vi "Inalfa SCU_Manual_LIN Message.vi"(0 "Choose Sequence":T1, 1 "LIN Device":T2={"Master Frame(3C)"="MasterReq\nSPA3414_ConfigurationsCMAGeely_CEMCALYPSOSDB34XX0Cfg_LIN3_190709_", "Slave Frame(3D)"="SlaveResp\nSPA3414_ConfigurationsCMAGeely_CEMCALYPSOSDB34XX0Cfg_LIN3_190709_", "Request Schedule"="CEMLIN3DiagRequestSchedule\nSPA3414_ConfigurationsCMAGeely_CEMCALYPSOSDB34XX0Cfg_LIN3_190709_", "Response Schedule"="CEMLIN3DiagResponseSchedule\nSPA3414_ConfigurationsCMAGeely_CEMCALYPSOSDB34XX0Cfg_LIN3_190709_", "Frame Write SCU"="", "Frame Read SCU"="", "LIN Name"=""}, 2 "Position":u16, 3 "Vent Cycles":u16, 4 "Slide Cycles":u16, 5 "Tx":u8[][](array[numeric]) format="%02x", 6 "Only Tx":u8[][](array[numeric]) format="%02x", 7 "Rx":u8[](array[numeric]) format="%02x", 8 "String":string, 10 "NAD":u8=36 format="%.0x") -> (11 "glass position":u16, 12 "TxRx Data":string[][](array[string]), 13 "sunshade position":u16, 14 "Response Good?":bool, 15 "Software Level":string, 16 "Hardware Level":string, 17 "Calfile Level":string, 18 "Glass Slide Cycle":u16, 19 "Rx2":u8[](array[numeric]) format="%02x")   [LabVIEW 2018]
uses:
  LIN Device.ctl
  LIN sequence for self SCU.ctl
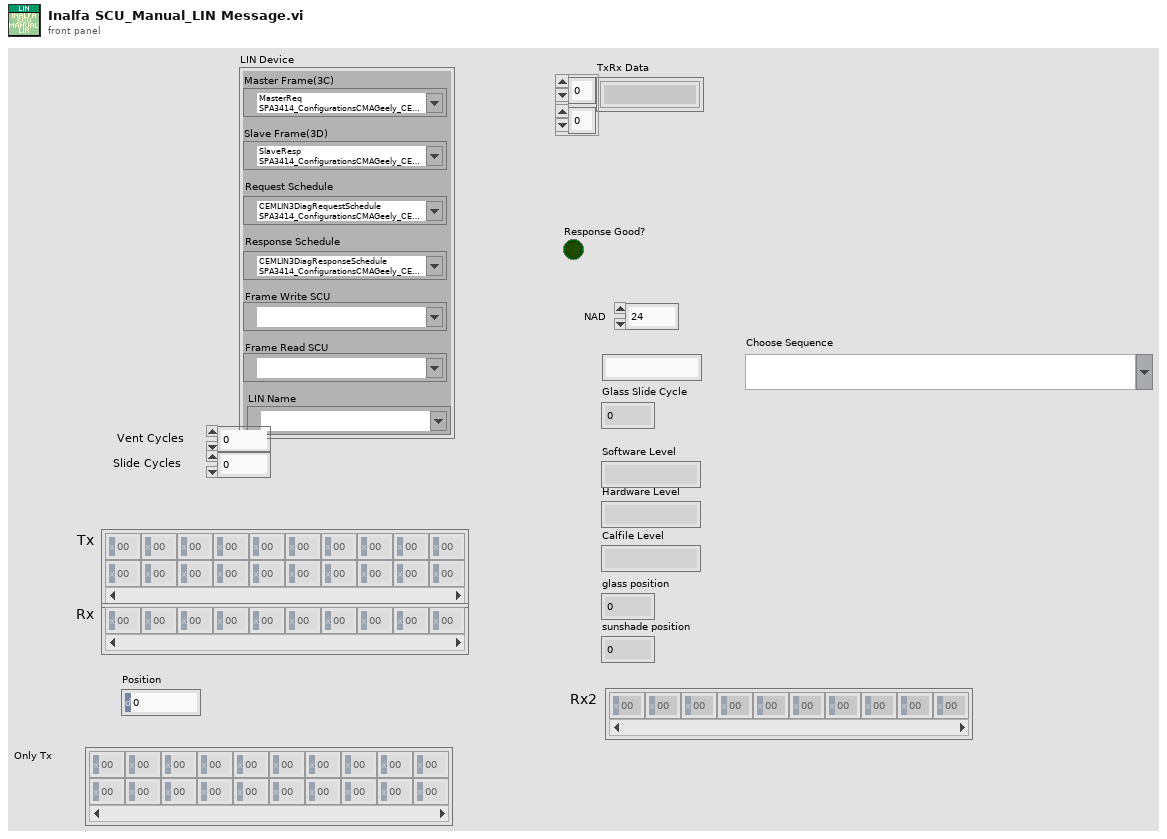
[diagram p1: front panel]
types:
  T1 = typedef "LIN sequence for self SCU.ctl" = string
  T2 = typedef "LIN Device.ctl" = cluster{"Master Frame(3C)":refnum<k21>, "Slave Frame(3D)":refnum<k21>, "Request Schedule":refnum<k21>, "Response Schedule":refnum<k21>, "Frame Write SCU":refnum<k21>, "Frame Read SCU":refnum<k21>, "LIN Name":refnum<k21>}
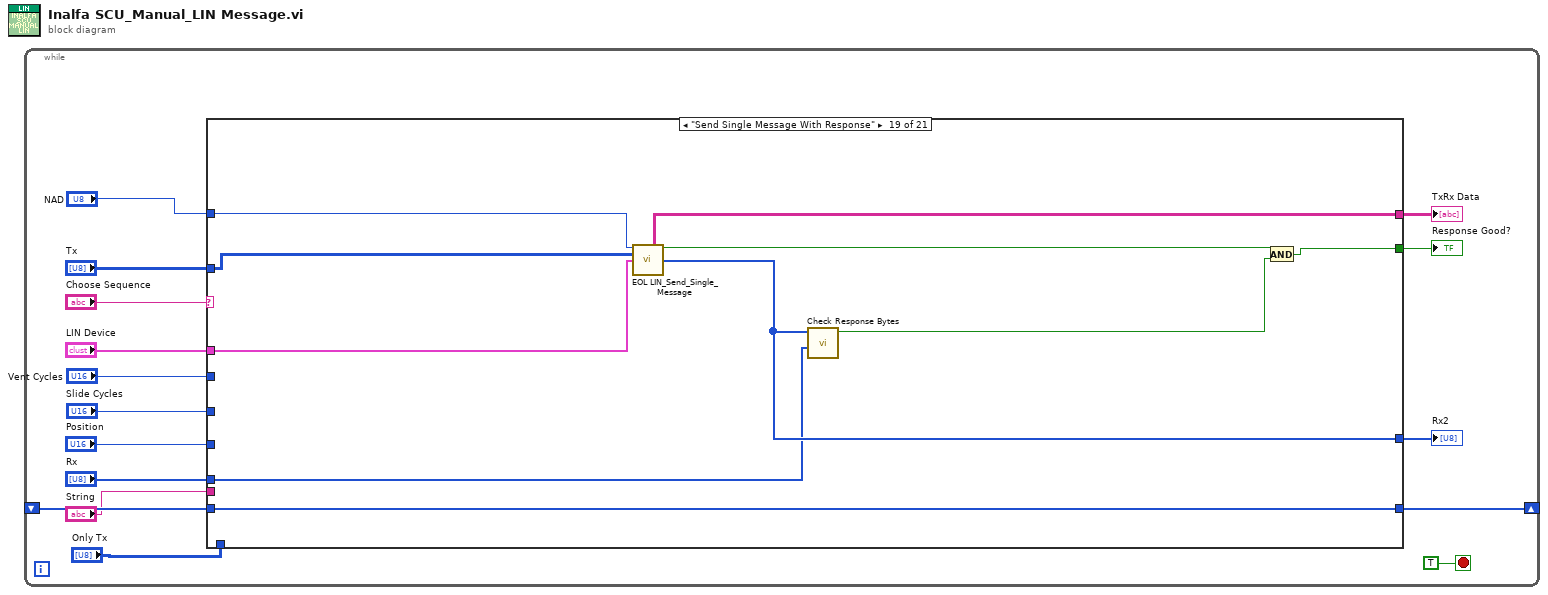
[diagram p0: block diagram]
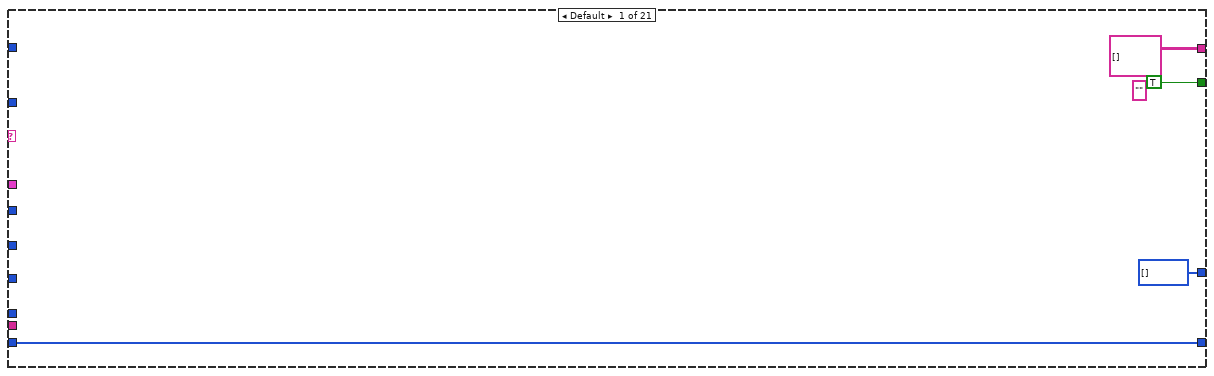
[diagram p2: hidden frame]
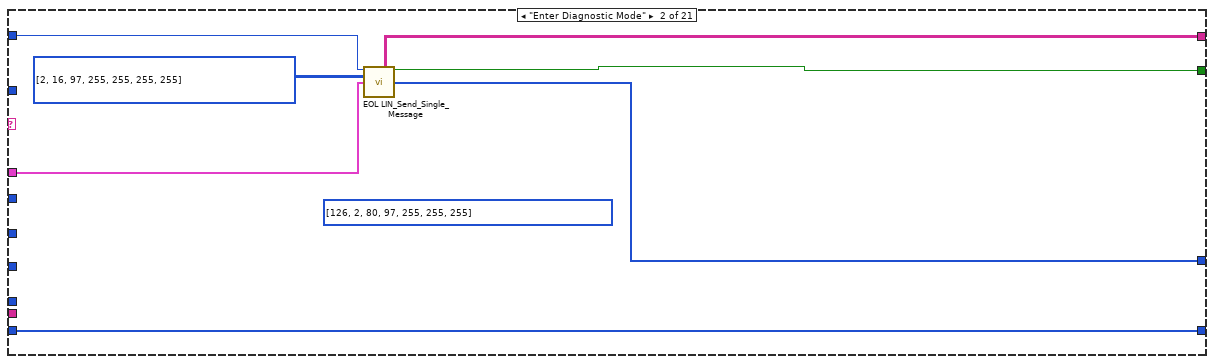
[diagram p3: hidden frame]
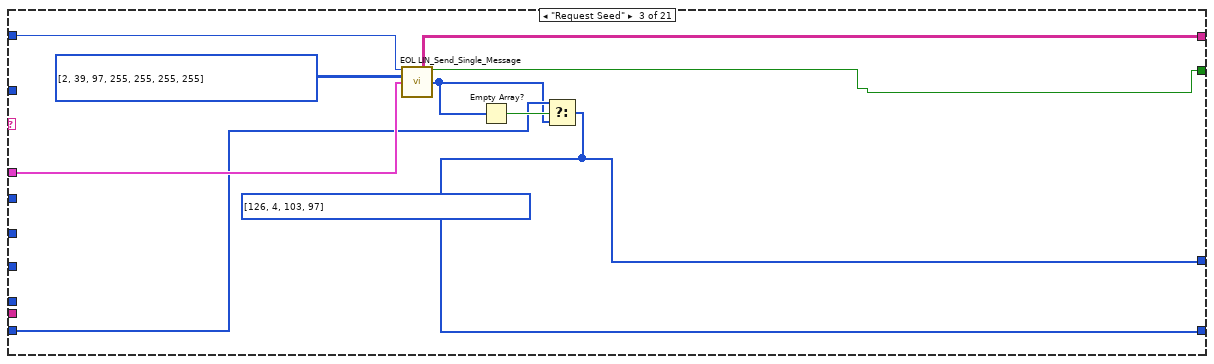
[diagram p4: hidden frame]
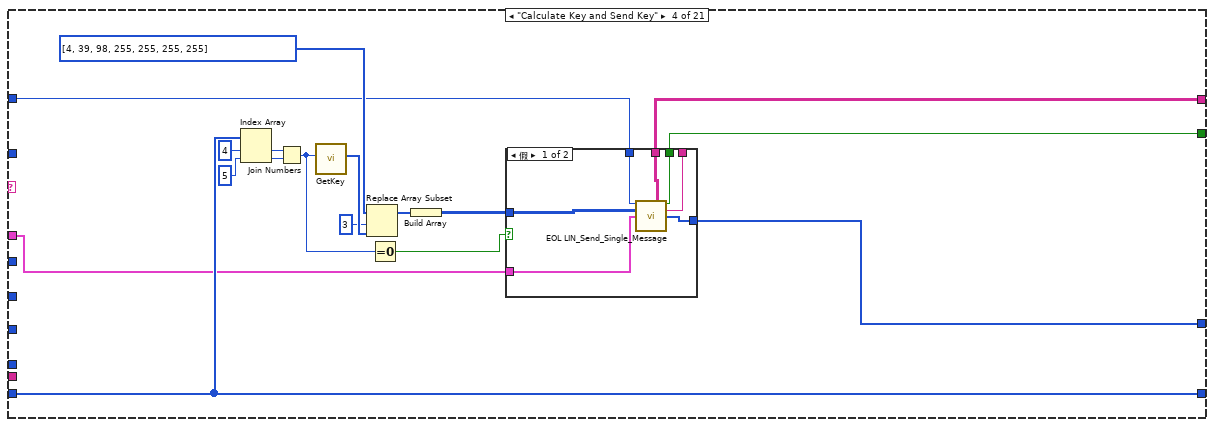
[diagram p5: hidden frame]
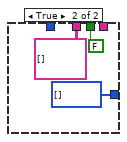
[diagram p6: hidden frame]
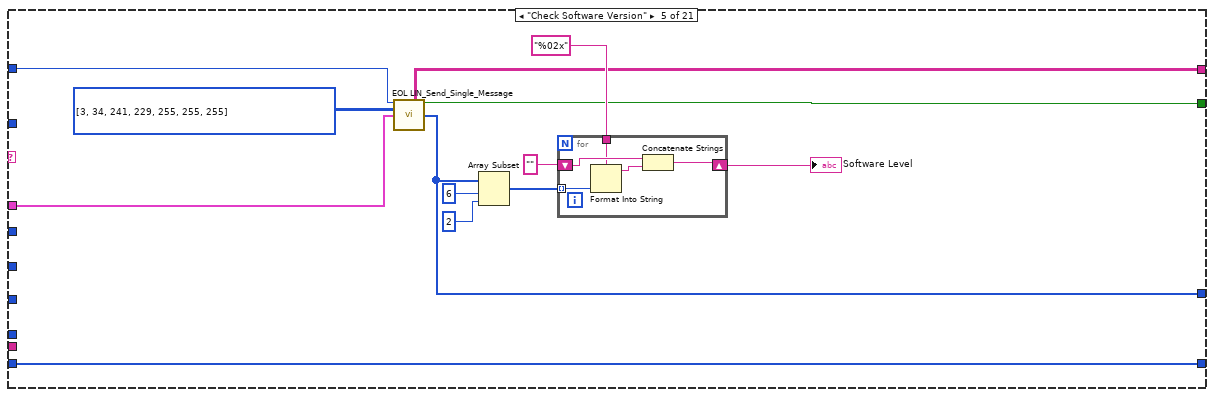
[diagram p7: hidden frame]
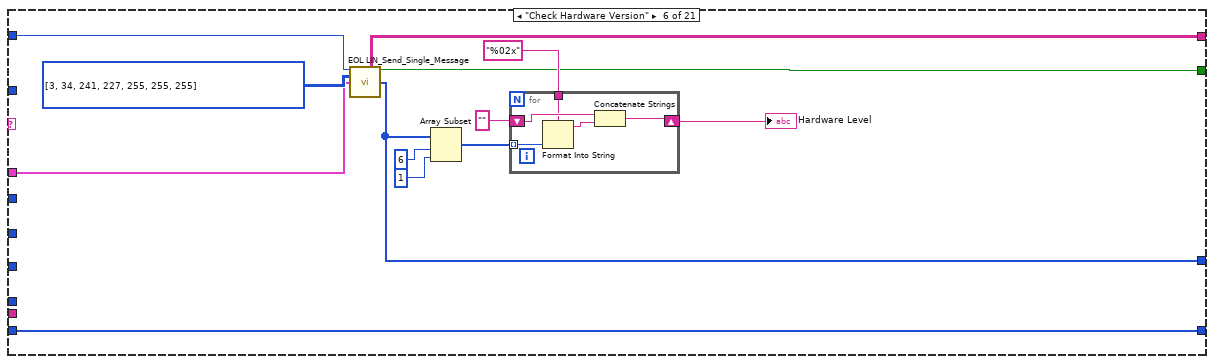
[diagram p8: hidden frame]
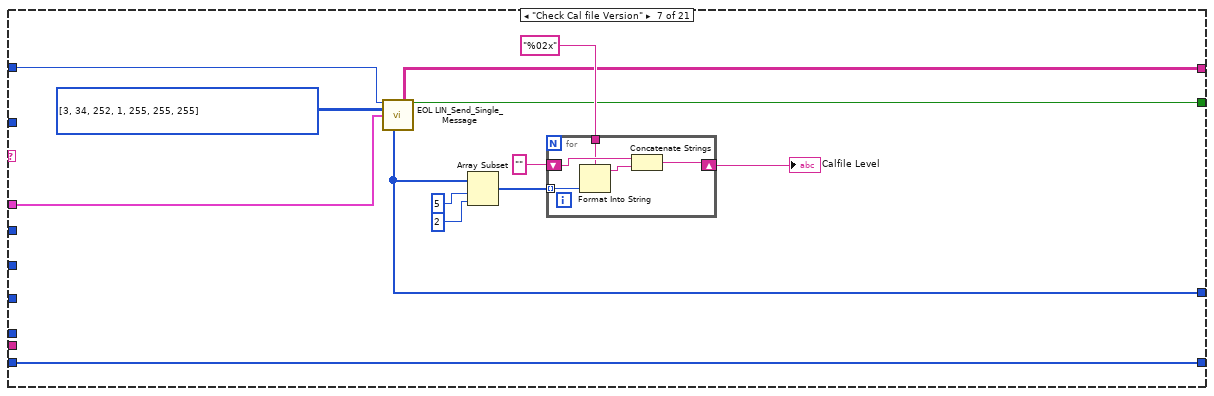
[diagram p9: hidden frame]
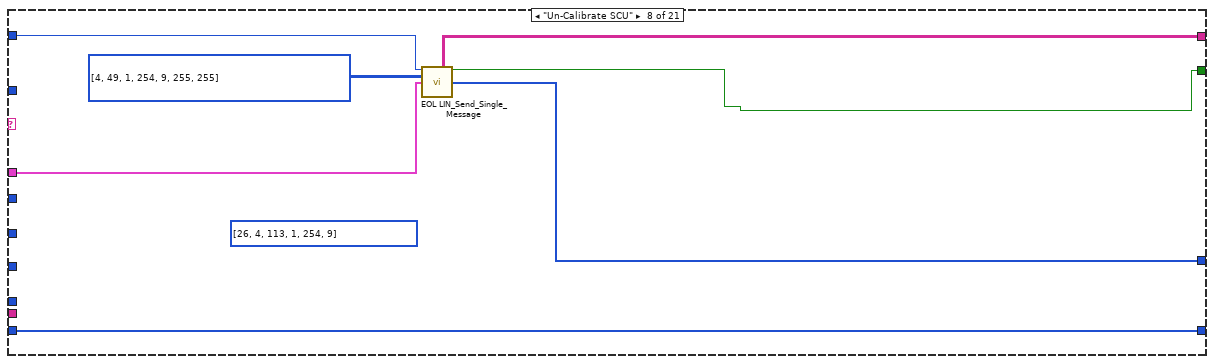
[diagram p10: hidden frame]
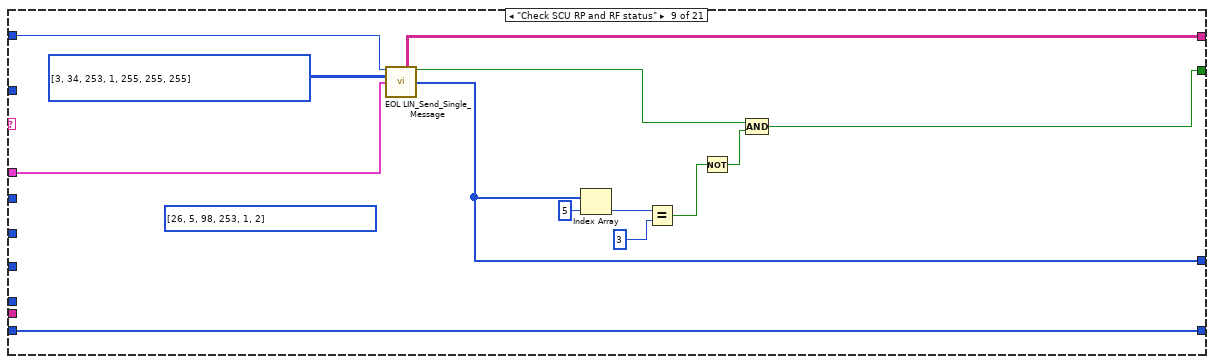
[diagram p11: hidden frame]
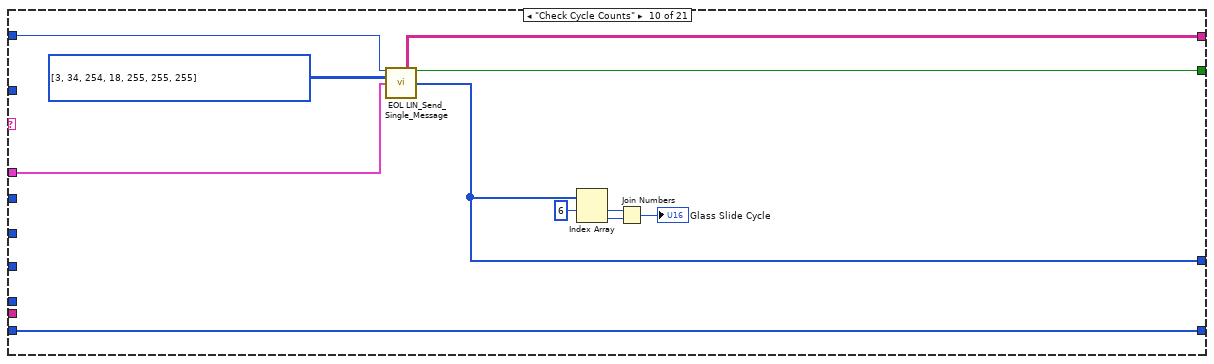
[diagram p12: hidden frame]
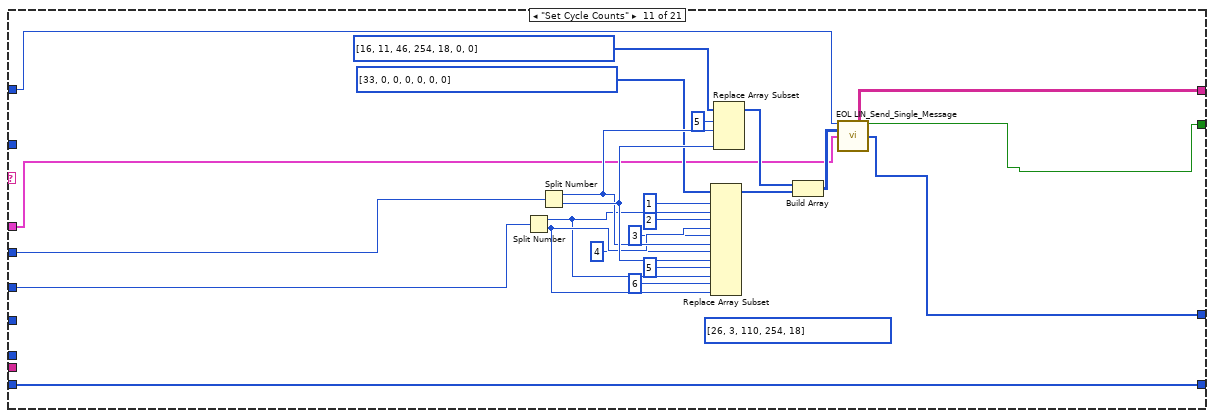
[diagram p13: hidden frame]
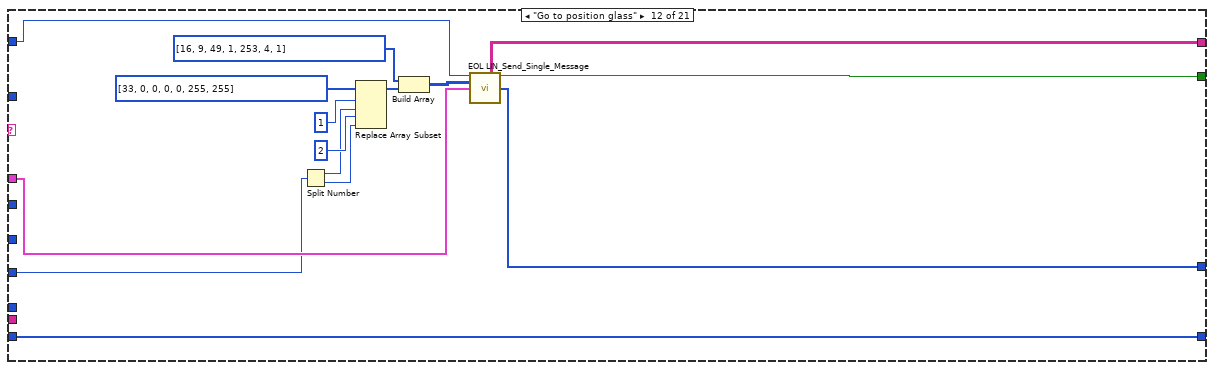
[diagram p14: hidden frame]
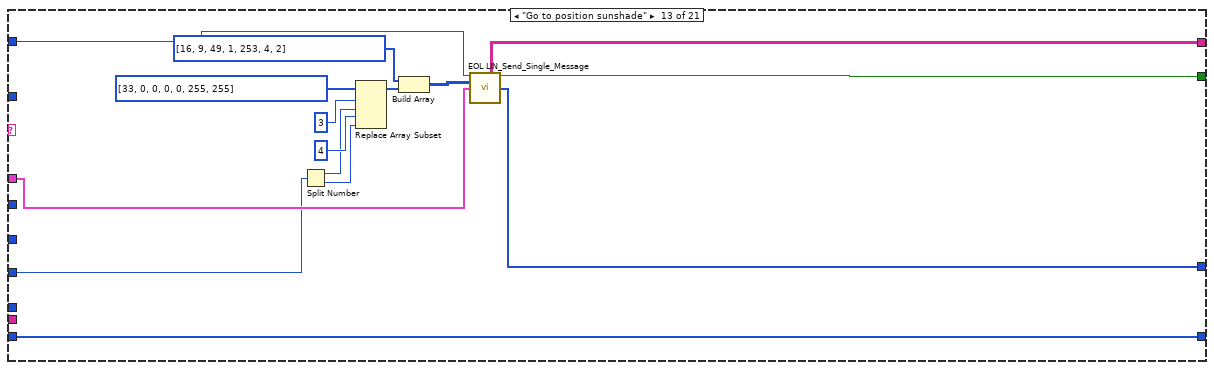
[diagram p15: hidden frame]
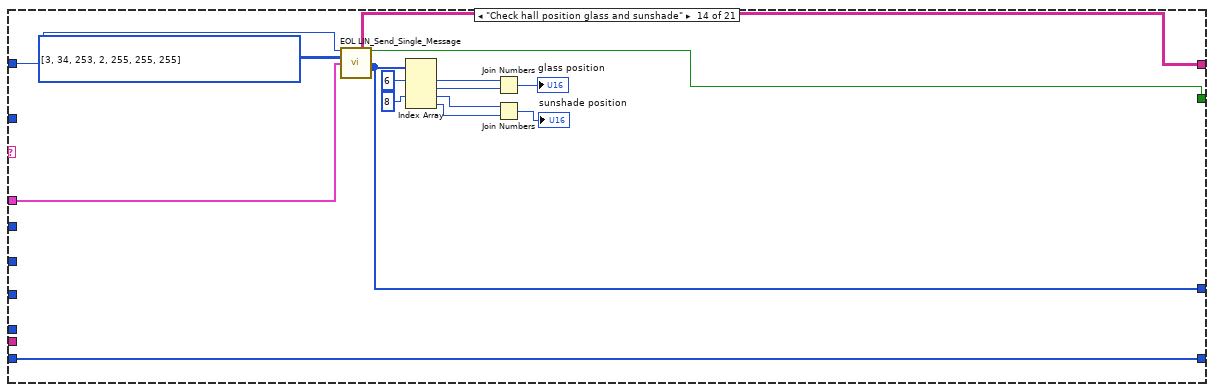
[diagram p16: hidden frame]
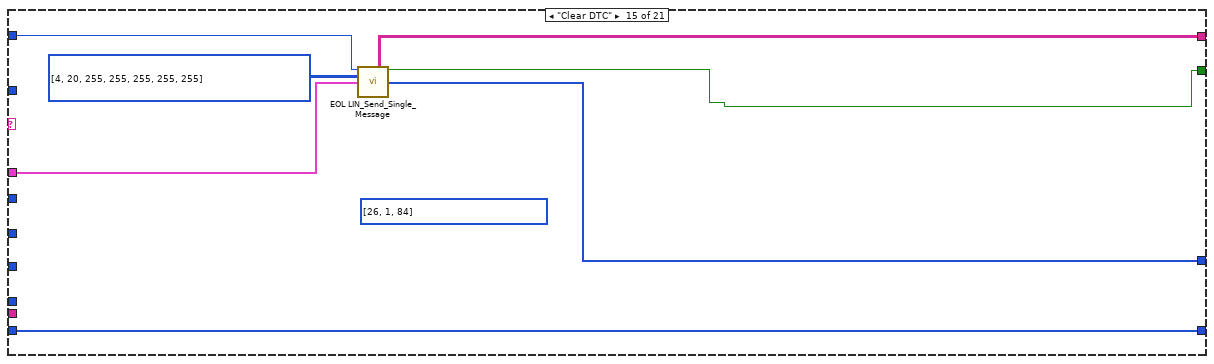
[diagram p17: hidden frame]
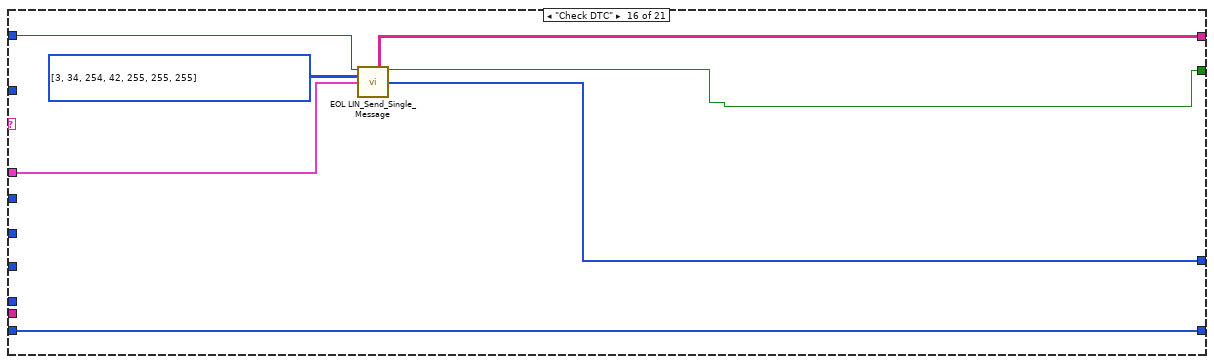
[diagram p18: hidden frame]
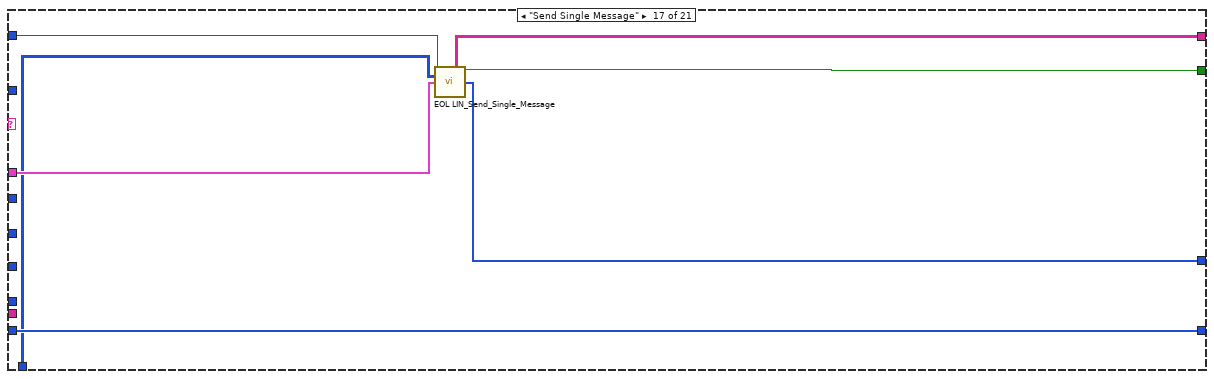
[diagram p19: hidden frame]
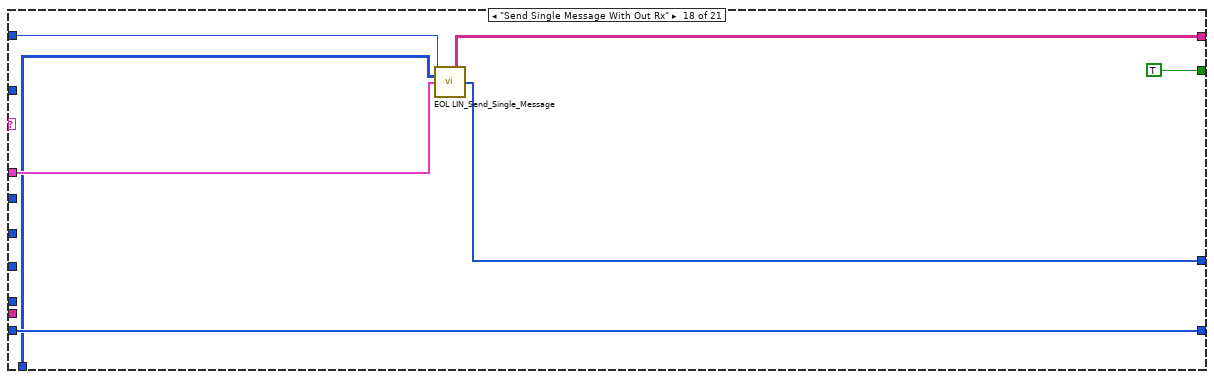
[diagram p20: hidden frame]
diagram:
  n1 = while {
    shift-right: [w12] -> _
    shift-left: _ -> [w11]
    stop <- TRUE stop-if-true
    n2 = case shown="\"Send Single Message With Response\"" "Choose Sequence" {
      tunnel: "LIN Device" -> [_ w26 w34 w39 w75 w87 w105 w123 w136 w147 w154 w176 w191 w208 w222 w229 w235 w242 w253 w265 w271]
      tunnel: [string[][] [] ("TxRx Data") w25 w35 w42 w69 w93 w107 w122 w135 w146 w156 w179 w194 w212 w223 w230 w238 w245 w255 w268 w274] -> w15
      tunnel: [TRUE ("Response Good?") w21 w28 w40 w65 w83 w101 w118 w132 w139 w149 w178 w193 w206 w218 w225 w237 TRUE ("Response Good?") w247 w267 w273] -> w14
      tunnel: [w18 w24 w31 w41 w68 w86 w104 w121 w134 w145 w155 w177 w192 w209 w221 w228 w236 w243 w254 w266 w272] -> w12
      tunnel: w11 -> [w18 w24 w32 w41 w68 w86 w104 w121 w134 w145 w155 w177 w192 w209 w221 w228 w236 w243 w254 w266 w272]
      tunnel: [u8[] [] ("Rx Message") w22 w31 w38 w67 w85 w103 w120 w126 w143 w153 w175 w190 w207 w220 w227 w234 w241 w251 w264 w270] -> w4
      tunnel: "Position" -> [_ _ _ _ _ _ _ _ _ _ _ w174 w189 _ _ _ _ _ _ _ _]
      tunnel: "Tx" -> [_ _ _ _ _ _ _ _ _ _ _ _ _ _ _ _ _ _ w252 _ _]
      tunnel: "Vent Cycles" -> [_ _ _ _ _ _ _ _ _ _ w152 _ _ _ _ _ _ _ _ _ _]
      tunnel: "Slide Cycles" -> [_ _ _ _ _ _ _ _ _ _ w151 _ _ _ _ _ _ _ _ _ _]
      tunnel: "Rx" -> [_ _ _ _ _ _ _ _ _ _ _ _ _ _ _ _ _ _ w250 _ _]
      tunnel: "Only Tx" -> [_ _ _ _ _ _ _ _ _ _ _ _ _ _ _ _ w233 w240 _ _ _]
      tunnel: "String" -> [_ _ _ _ _ _ _ _ _ _ _ _ _ _ _ _ _ _ _ w257 _]
      tunnel: "NAD" -> [_ w23 w29 w37 w64 w82 w100 w119 w125 w142 w150 w173 w188 w203 w219 w226 w232 w239 w246 w256 w269]
      frame Default {
        (unwired) "" ("spreadsheet string")
      }
      frame "Enter Diagnostic Mode" {
        (unwired) u8[] [126, 2, 80, 97, 255, 255, 255]
        n3 = call "EOL LIN_Send_Single_Message.vi"("NAD"=w23, "Tx Msg"=u8[][] [[2, 16, 97, 255, 255, 255, 255]], "LIN Device"=w26) -> ("TxRx Data"=w25:string[][], "Response Good?"=w21:bool, "Rx Msg"=w22:u8[])  [unwired: 8 in, 2 out]
      }
      frame "Request Seed" {
        (unwired) u8[] [126, 4, 103, 97]
        n4 = call "EOL LIN_Send_Single_Message.vi"("NAD"=w29, "Tx Msg"=u8[][] [[2, 39, 97, 255, 255, 255, 255]], "LIN Device"=w34) -> ("TxRx Data"=w35:string[][], "Response Good?"=w28:bool, "Rx Msg"=w30:u8[])  [unwired: 8 in, 2 out]
        n5 = Empty Array?(array=w30) -> (empty?=w33:bool)
        n6 = Select(t=w32, s=w33, f=w30) -> (s? t:f=w31:u8[])
      }
      frame "Calculate Key and Send Key" {
        n7 = Index Array(array=w41, index #1=4 ("index"), index #2=5 ("index")) -> (element #1=w51:u8, element #2=w50:u8)
        n8 = Join Numbers(hi=w51, lo=w50) -> ((hi.lo)=w45:u16)
        n9 = call "GetKey.vi"("x"=w45) -> ("KEY"=w49:u8[])  [unwired: 10 in]
        n10 = Replace Array Subset(array=u8[] [4, 39, 98, 255, 255, 255, 255], new element=w49, index=3) -> (w46:u8[])
        n11 = Equal To 0?(x=w45) -> (x = 0?=w43:bool)
        n12 = Build Array(w46) -> (w44:u8[][])
        n13 = case shown="假" w43 {
          tunnel: w44 -> [w60 _]
          tunnel: [w59 string[][] [] ("TxRx Data")] -> w42
          tunnel: [w58 FALSE ("Response Good?")] -> w40
          tunnel: [w57 _] -> _
          tunnel: w39 -> [w56 _]
          tunnel: [w55 u8[] [] ("Rx Message")] -> w38
          tunnel: w37 -> [w54 _]
          frame False {
            n14 = call "EOL LIN_Send_Single_Message.vi"("NAD"=w54, "Tx Msg"=w60, "LIN Device"=w56) -> ("TxRx Data"=w59:string[][], "Response Good?"=w58:bool, "spreadsheet string"=w57:string, "Rx Msg"=w55:u8[])  [unwired: 8 in, 1 out]
          }
          frame True {
          }
        }
      }
      frame "Check Software Version" {
        n15 = call "EOL LIN_Send_Single_Message.vi"("NAD"=w64, "Tx Msg"=u8[][] [[3, 34, 241, 229, 255, 255, 255]], "LIN Device"=w75) -> ("TxRx Data"=w69:string[][], "Response Good?"=w65:bool, "Rx Msg"=w67:u8[])  [unwired: 8 in, 2 out]
        n16 = Array Subset(array=w67, index=6, length=2) -> (w74:u8[])
        n17 = for {
          tunnel: w74 -> [w77] mode=indexing
          shift-right: [w80] -> w66
          shift-left: "" -> [w79]
          tunnel: "%02x" ("format string") -> [w78]
          n18 = Format Into String(format string=w78, w77) -> (resulting string=w81:string)  [unwired: 2 in, 1 out]
          n19 = Concatenate Strings(w79, w81) -> (w80:string)
        }
        "Software Level" <- w66
      }
      frame "Check Hardware Version" {
        n20 = call "EOL LIN_Send_Single_Message.vi"("NAD"=w82, "Tx Msg"=u8[][] [[3, 34, 241, 227, 255, 255, 255]], "LIN Device"=w87) -> ("TxRx Data"=w93:string[][], "Response Good?"=w83:bool, "Rx Msg"=w85:u8[])  [unwired: 8 in, 2 out]
        n21 = Array Subset(array=w85, index=6, length=1) -> (w92:u8[])
        n22 = for {
          tunnel: w92 -> [w95] mode=indexing
          shift-right: [w98] -> w84
          shift-left: "" -> [w97]
          tunnel: "%02x" ("format string") -> [w96]
          n23 = Format Into String(format string=w96, w95) -> (resulting string=w99:string)  [unwired: 2 in, 1 out]
          n24 = Concatenate Strings(w97, w99) -> (w98:string)
        }
        "Hardware Level" <- w84
      }
      frame "Check Cal file Version" {
        n25 = call "EOL LIN_Send_Single_Message.vi"("NAD"=w100, "Tx Msg"=u8[][] [[3, 34, 252, 1, 255, 255, 255]], "LIN Device"=w105) -> ("TxRx Data"=w107:string[][], "Response Good?"=w101:bool, "Rx Msg"=w103:u8[])  [unwired: 8 in, 2 out]
        n26 = Array Subset(array=w103, index=5, length=2) -> (w112:u8[])
        n27 = for {
          tunnel: w112 -> [w113] mode=indexing
          shift-right: [w116] -> w102
          shift-left: "" -> [w115]
          tunnel: "%02x" ("format string") -> [w114]
          n28 = Format Into String(format string=w114, w113) -> (resulting string=w117:string)  [unwired: 2 in, 1 out]
          n29 = Concatenate Strings(w115, w117) -> (w116:string)
        }
        "Calfile Level" <- w102
      }
      frame "Un-Calibrate SCU" {
        (unwired) u8[] [26, 4, 113, 1, 254, 9]
        n30 = call "EOL LIN_Send_Single_Message.vi"("NAD"=w119, "Tx Msg"=u8[][] [[4, 49, 1, 254, 9, 255, 255]], "LIN Device"=w123) -> ("TxRx Data"=w122:string[][], "Response Good?"=w118:bool, "Rx Msg"=w120:u8[])  [unwired: 8 in, 2 out]
      }
      frame "Check SCU RP and RF status" {
        (unwired) u8[] [26, 5, 98, 253, 1, 2]
        n31 = call "EOL LIN_Send_Single_Message.vi"("NAD"=w125, "Tx Msg"=u8[][] [[3, 34, 253, 1, 255, 255, 255]], "LIN Device"=w136) -> ("TxRx Data"=w135:string[][], "Response Good?"=w133:bool, "Rx Msg"=w126:u8[])  [unwired: 8 in, 2 out]
        n32 = Index Array(array=w126, index=5) -> (element=w130:u8)
        n33 = Equal?(x=w130, y=u8 3 ("element")) -> (x = y?=w128:bool)
        n34 = Not(x=w128) -> (.not. x?=w127:bool)
        n35 = Compound Arithmetic op=AND(w133, w127) -> (w132:bool)
      }
      frame "Check Cycle Counts" {
        n36 = call "EOL LIN_Send_Single_Message.vi"("NAD"=w142, "Tx Msg"=u8[][] [[3, 34, 254, 18, 255, 255, 255]], "LIN Device"=w147) -> ("TxRx Data"=w146:string[][], "Response Good?"=w139:bool, "Rx Msg"=w143:u8[])  [unwired: 8 in, 2 out]
        n37 = Index Array(array=w143, index #1=6 ("index")) -> (element #1=w141:u8, element #2=w140:u8)  [unwired: 1 in]
        n38 = Join Numbers(hi=w141, lo=w140) -> ((hi.lo)=→"Glass Slide Cycle":u16)
      }
      frame "Set Cycle Counts" {
        (unwired) u8[] [26, 3, 110, 254, 18]
        n39 = Split Number(x=w151) -> (hi(x)=w167:u8, lo(x)=w168:u8)
        n40 = Split Number(x=w152) -> (hi(x)=w169:u8, lo(x)=w170:u8)
        n41 = Replace Array Subset(array=u8[] [33, 0, 0, 0, 0, 0, 0] ("Frame payloads to queue"), new element #1=w167, index #1=1 ("索引"), new element #2=w168, index #2=2 ("索引"), new element #3=w169, index #3=3 ("索引"), new element #4=w170, index #4=4 ("索引"), new element #5=w167, index #5=5 ("索引"), new element #6=w168, index #6=6 ("索引")) -> (w172:u8[])
        n42 = Replace Array Subset(array=u8[] [16, 11, 46, 254, 18, 0, 0] ("Frame payloads to queue"), new element #1=w169, index #1=5 ("索引"), new element #2=w170) -> (w171:u8[])  [unwired: 1 in]
        n43 = Build Array(w171, w172) -> (w157:u8[][])
        n44 = call "EOL LIN_Send_Single_Message.vi"("NAD"=w150, "Tx Msg"=w157, "LIN Device"=w154) -> ("TxRx Data"=w156:string[][], "Response Good?"=w149:bool, "Rx Msg"=w153:u8[])  [unwired: 8 in, 2 out]
      }
      frame "Go to position glass" {
        n45 = Split Number(x=w174) -> (hi(x)=w185:u8, lo(x)=w184:u8)
        n46 = Replace Array Subset(array=u8[] [33, 0, 0, 0, 0, 255, 255], new element #1=w185, index #1=1 ("index"), new element #2=w184, index #2=2 ("index")) -> (w182:u8[])
        n47 = Build Array(u8[] [16, 9, 49, 1, 253, 4, 1], w182) -> (w180:u8[][])
        n48 = call "EOL LIN_Send_Single_Message.vi"("NAD"=w173, "Tx Msg"=w180, "LIN Device"=w176) -> ("TxRx Data"=w179:string[][], "Response Good?"=w178:bool, "Rx Msg"=w175:u8[])  [unwired: 8 in, 2 out]
      }
      frame "Go to position sunshade" {
        n49 = Split Number(x=w189) -> (hi(x)=w200:u8, lo(x)=w199:u8)
        n50 = Replace Array Subset(array=u8[] [33, 0, 0, 0, 0, 255, 255], new element #1=w200, index #1=3 ("index"), new element #2=w199, index #2=4 ("index")) -> (w197:u8[])
        n51 = Build Array(u8[] [16, 9, 49, 1, 253, 4, 2], w197) -> (w195:u8[][])
        n52 = call "EOL LIN_Send_Single_Message.vi"("NAD"=w188, "Tx Msg"=w195, "LIN Device"=w191) -> ("TxRx Data"=w194:string[][], "Response Good?"=w193:bool, "Rx Msg"=w190:u8[])  [unwired: 8 in, 2 out]
      }
      frame "Check hall position glass and sunshade" {
        n53 = call "EOL LIN_Send_Single_Message.vi"("NAD"=w203, "Tx Msg"=u8[][] [[3, 34, 253, 2, 255, 255, 255]], "LIN Device"=w208) -> ("TxRx Data"=w212:string[][], "Response Good?"=w206:bool, "Rx Msg"=w207:u8[])  [unwired: 8 in, 2 out]
        n54 = Index Array(array=w207, index #1=6 ("index"), index #3=8 ("index")) -> (element #1=w215:u8, element #2=w214:u8, element #3=w211:u8, element #4=w210:u8)  [unwired: 2 in]
        n55 = Join Numbers(hi=w215, lo=w214) -> ((hi.lo)=→"glass position":u16)
        n56 = Join Numbers(hi=w211, lo=w210) -> ((hi.lo)=→"sunshade position":u16)
      }
      frame "Clear DTC" {
        (unwired) u8[] [26, 1, 84]
        n57 = call "EOL LIN_Send_Single_Message.vi"("NAD"=w219, "Tx Msg"=u8[][] [[4, 20, 255, 255, 255, 255, 255]], "LIN Device"=w222) -> ("TxRx Data"=w223:string[][], "Response Good?"=w218:bool, "Rx Msg"=w220:u8[])  [unwired: 8 in, 2 out]
      }
      frame "Check DTC" {
        n58 = call "EOL LIN_Send_Single_Message.vi"("NAD"=w226, "Tx Msg"=u8[][] [[3, 34, 254, 42, 255, 255, 255]], "LIN Device"=w229) -> ("TxRx Data"=w230:string[][], "Response Good?"=w225:bool, "Rx Msg"=w227:u8[])  [unwired: 8 in, 2 out]
      }
      frame "Send Single Message" {
        n59 = call "EOL LIN_Send_Single_Message.vi"("NAD"=w232, "Tx Msg"=w233, "LIN Device"=w235) -> ("TxRx Data"=w238:string[][], "Response Good?"=w237:bool, "Rx Msg"=w234:u8[])  [unwired: 8 in, 2 out]
      }
      frame "Send Single Message With Out Rx" {
        n60 = call "EOL LIN_Send_Single_Message.vi"("NAD"=w239, "Tx Msg"=w240, "LIN Device"=w242) -> ("TxRx Data"=w245:string[][], "Rx Msg"=w241:u8[])  [unwired: 8 in, 3 out]
      }
      frame "Send Single Message With Response" {
        n61 = call "EOL LIN_Send_Single_Message.vi"("NAD"=w246, "Tx Msg"=w252, "LIN Device"=w253) -> ("TxRx Data"=w255:string[][], "Response Good?"=w249:bool, "Rx Msg"=w251:u8[])  [unwired: 8 in, 2 out]
        n62 = call "Check Response Bytes.vi"("Data Bytes"=w250, "Response Bytes"=w251) -> ("Pass?"=w248:bool)  [unwired: 9 in]
        n63 = And(x=w249, y=w248) -> (x .and. y?=w247:bool)
      }
      frame "Inalfa SCU Teach" {
        n64 = Decimal String To Number(string=w257, default (0L)=u8 0) -> (number=w259:u8)  [unwired: 1 in, 1 out]
        n65 = Replace Array Subset(array=u8[][] [[5, 49, 1, 240, 0, 3, 255]], new element=w259, index (row)=0, index (col)=5 ("disabled index (col)")) -> (w258:u8[][])
        n66 = call "EOL LIN_Send_Single_Message.vi"("NAD"=w256, "Tx Msg"=w258, "LIN Device"=w265) -> ("TxRx Data"=w268:string[][], "Response Good?"=w267:bool, "Rx Msg"=w264:u8[])  [unwired: 8 in, 2 out]
      }
      frame "Hold EOL session" {
        n67 = call "EOL LIN_Send_Single_Message.vi"("NAD"=w269, "Tx Msg"=u8[][] [[2, 62, 0, 255, 255, 255, 255]], "LIN Device"=w271) -> ("TxRx Data"=w274:string[][], "Response Good?"=w273:bool, "Rx Msg"=w270:u8[])  [unwired: 8 in, 2 out]
      }
    }
    "TxRx Data" <- w15
    "Response Good?" <- w14
    "Rx2" <- w4
  }
